vi "SPC_close.vi"(8 "Error In":errorcluster, 11 "DLL Path":path) -> (0 "Error Out":errorcluster, 3 "DLL Path":path)   [LabVIEW 2019]
doc: "The procedure frees buffers allocated via DLL and set the DLL state as before SPC_init call.\nSPC_init is the only procedure which can be called after SPC_close.\n\ninfo@becker-hickl.com"
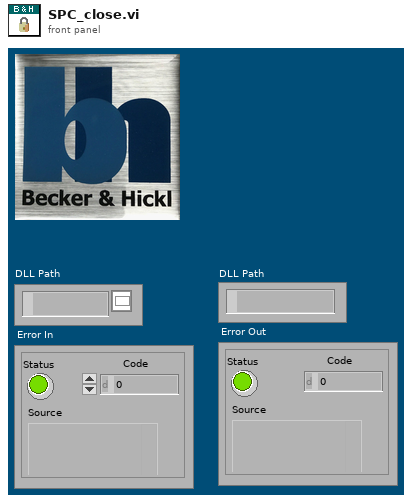
[diagram p1: front panel]
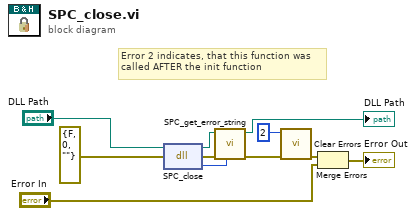
[diagram p0: block diagram]
diagram:
  # "Error 2 indicates, that this function was\ncalled AFTER the init function"
  n1 = dll-call lib="D:/spcm/lib/lab_view/lv10.0/spcm32.dll" fn="SPC_close"(path in="DLL Path", error in=errorcluster {"status"=FALSE, "code"=0, "source"=""} ("error constant")) -> (path out=w4:path, error out=w6:errorcluster, "return type"=w7:i16)  [unwired: 1 in]
  n2 = call "SPC_get_error_string.vi"("ErrorID"=w7, "Error In"=w6, "DLL Path"=w4) -> ("Error Out"=w5:errorcluster, "DLL Path"=→"DLL Path":path)  [unwired: 6 in, 1 out]
  n3 = call <vilib>:"Clear Errors.vi"("error in (no error)"=w5, "specific error code to clear (0: all)"=2) -> ("error out"=w9:errorcluster)  [unwired: 4 in, 1 out]
  n4 = Merge Errors(w9, "Error In") -> (→"Error Out":errorcluster)
